vi "Grips Slave UDP (PXI).vi"() -> ()   [LabVIEW 2013]
uses:
  <vilib>/Analysis/Matrix/Datatypes/RealMatrix.ctl
  Telemanipulation/PXI/PXI.lvclass
  Telemanipulation/Grips Robot/Grips Robot.lvclass
  <vilib>/Platform/TimedLoop/XDataNode/timing_clust.ctl
  <vilib>/Platform/TimedLoop/XDataNode/nitl_modes.ctl
  <vilib>/Platform/TimedLoop/XDataNode/wakeup.ctl
  labview_ros/sensor_msgs/JointState.ctl
  labview_ros/std_msgs/Header.ctl
  Telemanipulation/Grips Robot/Grips Robot.lvclass/Grips Robot.ctl
  Telemanipulation/Hardware Interface/Hardware Interface.lvclass/Hardware Interface.ctl
  labview_ros/osrf_msgs/JointCommands.ctl
  Telemanipulation/Hardware Interface/Set HW Interface Analog Outputs.vi
  <userlib>/_matio/level5/Public/Write/Append Data Element.llb/Append Data Element (1D Array of Double).vi
  <userlib>/_matio/level5/Public/Write/Append Data Element.llb/Append Data Element (2D Array of Double).vi
  Telemanipulation/Helpers/Order JointCommands By Name.vi
  <vilib>/addons/control/pid/pid.llb/PID.vi
  <vilib>/addons/control/pid/pid.llb/PID (DBL).vi
  <vilib>/Platform/TimedLoop/XDataNode/XDataNode.xnode
  <vilib>/Platform/TimedLoop/XDataNode/XDNodeRunTimeDep.lvlib
  Telemanipulation/Helpers/Helpers.lvlib
  <userlib>/_matio/level5.lvlib
  <vilib>/Analysis/Matrix/NI_Matrix.lvlib
panel:
  out "end effector transform":T1
  in  "Data Logging":cluster{"Path":path, "Save":bool}={"Path"=path "c:/ni-rt/testing/slave_udp.mat", "Save"=FALSE}
  out "Logging Status":errorcluster
  out "UDP Receiver":cluster{"Rate (Hz)":dbl, "Status":errorcluster}
  out "UDP Sender":cluster{"Rate (Hz)":dbl, "Status":errorcluster}
  out "Joint Names":string[](array[string])=["SA", "SE", "EL", "WP", "WY", "WR"]
  in  "ROS Machine":T2={"IP"="192.168.0.10", "Read Port"=5051, "Write Port"=5052}
  out "WR":dbl(slide)=-0.9473827382931216 scale=-3.14..3.14
  out "WY":dbl(slide)=0.3565705572681916 scale=-1.01..0.67
  out "WP":dbl(slide)=-0.29450757439331093 scale=-1.1..0.58
  out "EL":dbl(slide)=3.229844911017393 scale=0.74..4.2
  out "SE":dbl(slide)=-1.3453457540222367 scale=-1.5..0.5
  out "SA":dbl(slide)=0.31900452488687786 scale=-1.5..1.5
  in  "Hyd ON":bool
  in  "kp_position":dbl[](array[numeric])=[3.0, -1.5, 2.0, 4.0, -2.0, 4.0]
  in  "stop":bool
  out "System Status":errorcluster
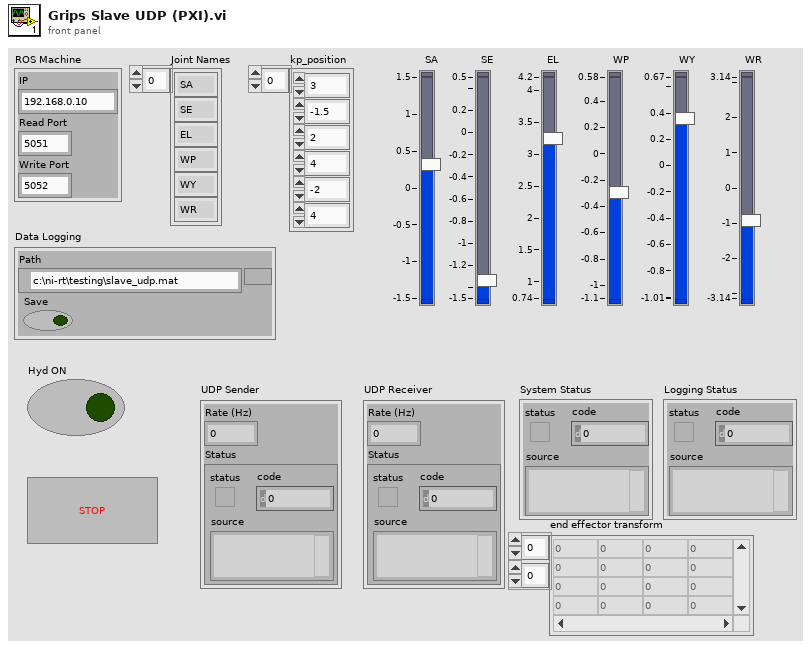
[diagram p1: front panel]
types:
  T1 = typedef "NI_Matrix.lvlib/RealMatrix.ctl" = dbl[][]
  T2 = cluster{"IP":string, "Read Port":u16, "Write Port":u16}
  T3 = typedef "XDNodeRunTimeDep.lvlib/timing_clust.ctl" = cluster{"Expected End [f-1]":u64, "Actual End [f-1]":u64, "Finished Late? [f-1]":bool, "Expected End [i-1]":u64, "Actual End [i-1]":u64, "Finished Late? [i-1]":bool, "Expected Start [i]":u64, "Actual Start [i]":u64, "Expected Start [f]":u64, "Actual Start [f]":u64, "Source Name":string, "Structure Name":string, "Period":i64, "Deadline":i64, "Offset":i64, "Start":i64, "Priority":i32, "Timeout":i32, "Mode":T4, "Wakeup Reason":T5, "Error":errorcluster, "Source Type":string, "Secondary Source Type":string, "Global End Time":u64, "Global Start Time":u64, "Frame Duration":u64, "Iteration Duration":u64, "Assigned CPU":i32, "I/O Scan Engine Mode":u32}
  T4 = typedef "XDNodeRunTimeDep.lvlib/nitl_modes.ctl" = enum32{"No Change", "Process missed periods, maintain original phase", "Discard missed periods, maintain original phase", "Process missed periods, ignore original phase", "Discard missed periods, ignore original phase"}
  T5 = typedef "XDNodeRunTimeDep.lvlib/wakeup.ctl" = enum32{"Normal", "Aborted", "Asynchronous wakeup", "Timing source error", "Timed loop error", "Timeout"}
  T6 = typedef "Grips Robot.lvclass/JointMapping.ctl" = cluster{"name":string[], "position":string[], "velocity":string[], "effort":string[], "command":string[]}
  T7 = cluster{"names":cluster{"AI":string[], "AO":string[], "DI":string[], "DO":string[]}, "interpolation_coeff":sgl[][]}
  T8 = typedef "NI_Robotics_Link.lvclass/Joint Type.ctl" = enum16{"Revolute", "Prismatic"}
  T9 = cluster{"k":sgl[][], "p":sgl[][], "T0":sgl[][], "types":T8[], "joint_limits":cluster{"has_limits":bool[], "min_position":sgl[], "max_position":sgl[]}}
  T10 = enum16{"big-endian, network order", "native, host order", "little-endian"}
  T11 = typedef "JointState.ctl" = cluster{"header":T12, "name":string[], "position":dbl[], "velocity":dbl[], "effort":dbl[]}
  T12 = typedef "Header.ctl" = cluster{"seq":u32, "stamp":cluster{"sec":i32, "nsec":i32}, "frame_id":string}
  T13 = cluster{"seq":u32, "stamp":cluster{"sec":i32, "nsec":i32}, "frame_id":string}
  T14 = cluster{"AI":string[], "AO":string[], "DI":string[], "DO":string[]}
  T15 = typedef "PXI.lvclass/Task Definition.ctl" = cluster{"task_type":T16, "names":string[], "physical channels":tag, "min_value":dbl, "max_value":dbl, "task_number":i32}
  T16 = typedef "PXI.lvclass/Task Types.ctl" = enum16{"Analog Input", "Analog Output", "Digital Input", "Digital Output"}
  T17 = enum16{"open", "replace", "create", "open or create", "replace or create", "replace or create with confirmation"}
  T18 = typedef "Hardware Interface.lvclass/BoolArrayWithName.ctl" = cluster{"name":string[], "value":bool[]}
  T19 = typedef "Hardware Interface.lvclass/DblArrayWithName.ctl" = cluster{"name":string[], "value":dbl[]}
  T20 = typedef "JointCommands.ctl" = cluster{"header":T12, "name":string[], "position":dbl[], "velocity":dbl[], "effort":dbl[], "kp_position":dbl[], "ki_position":dbl[], "kd_position":dbl[], "kp_velocity":dbl[], "i_effort_min":dbl[], "i_effort_max":dbl[]}
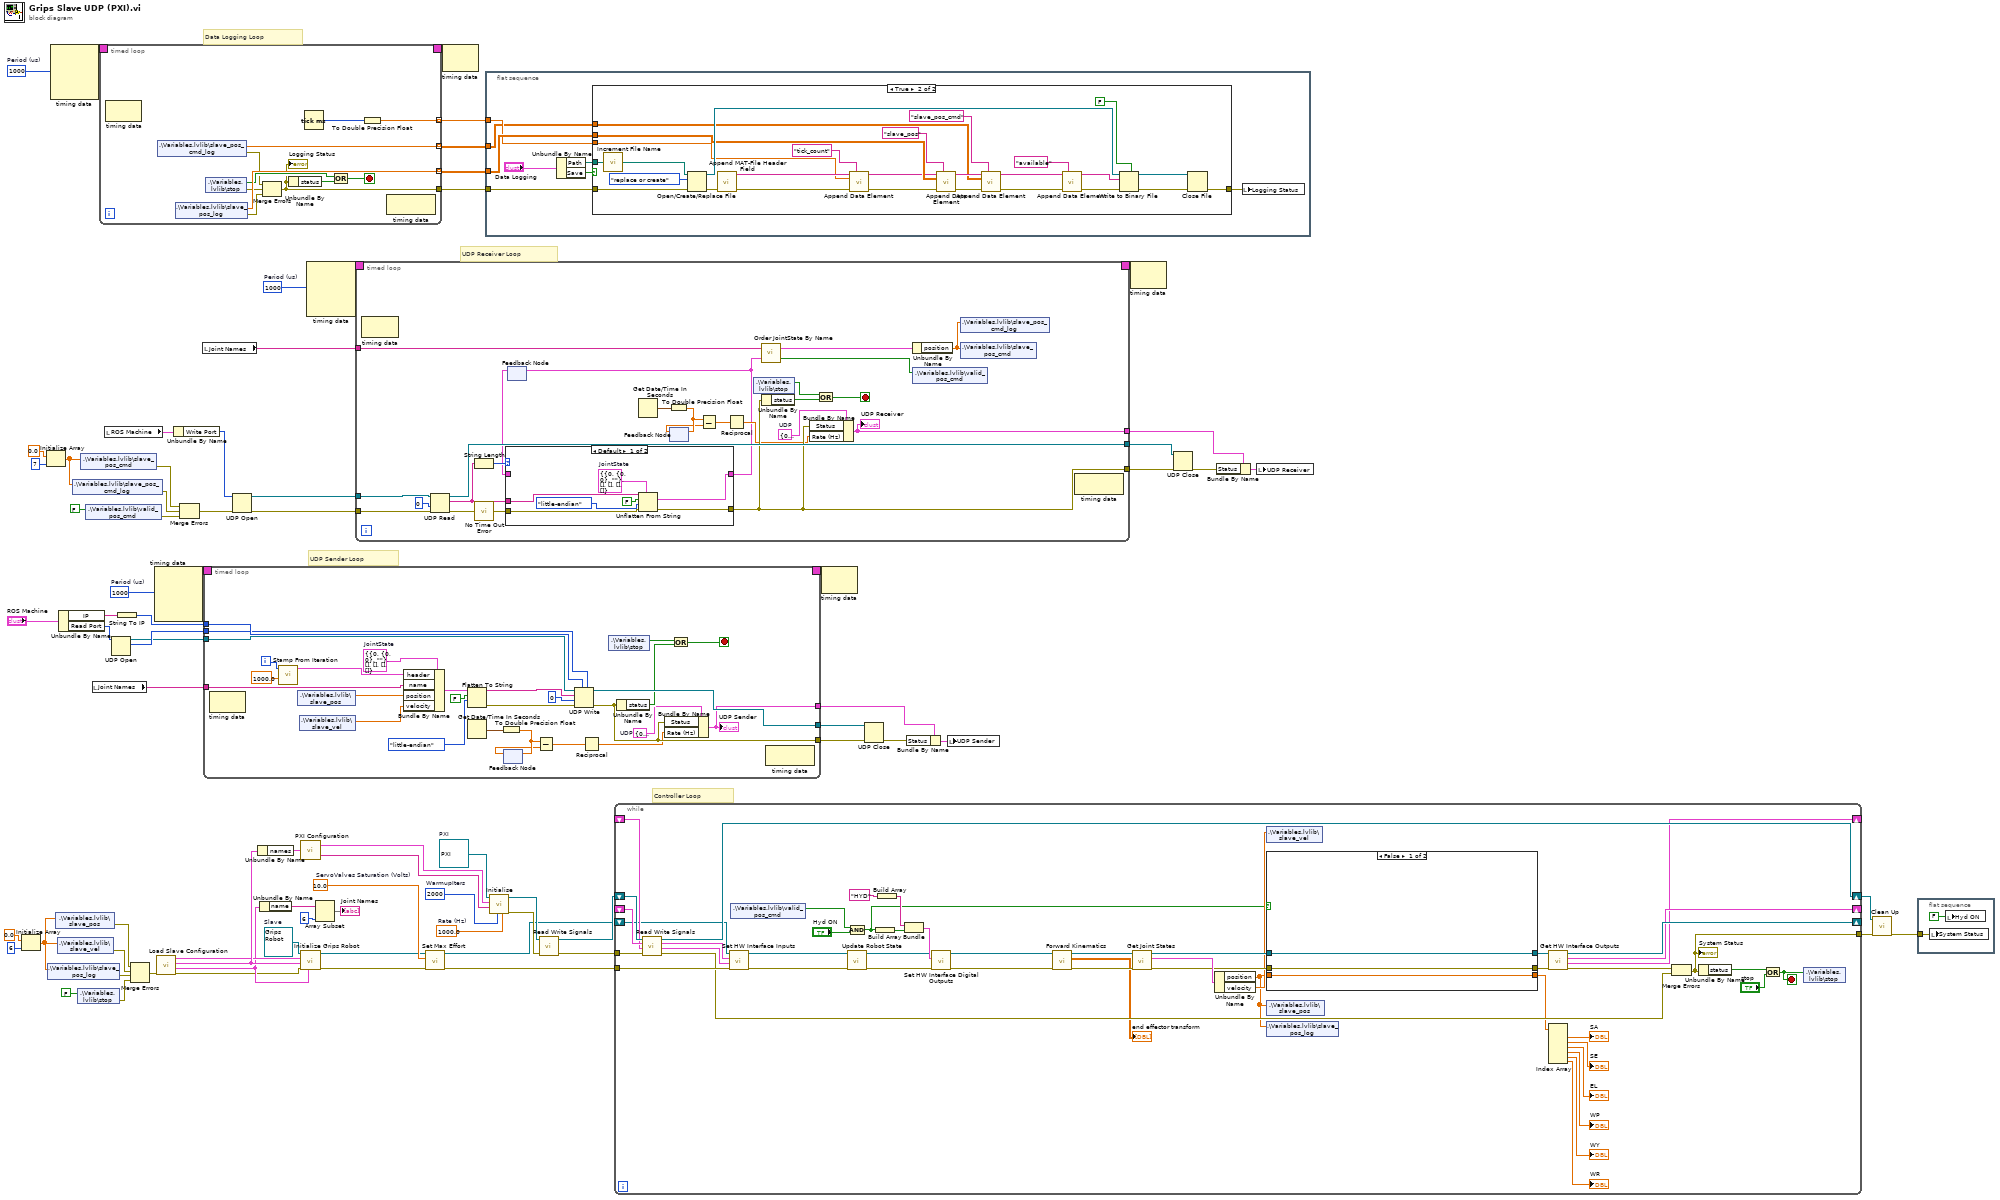
[diagram p0: block diagram]
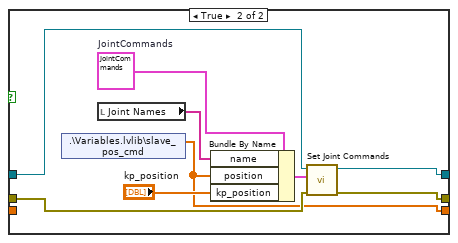
[diagram p4: hidden frame]
diagram:
  w5 = i64 1000  # Period (us)
  w30 = i64 1000  # Period (us)
  w49 = i64 1000  # Period (us)
  w62 = 10.0  # ServoValves Saturation (Volts)
  w65 = refnum<class "Grips Robot.lvclass"> refnum  # Slave
  w76 = 1000.0  # Rate (Hz)
  w77 = u32 2000  # WarmupIters
  w78 = refnum<class "PXI.lvclass"> refnum  # PXI
  # "Data Logging Loop"
  # "Controller Loop"
  # "UDP Receiver Loop"
  # "UDP Sender Loop"
  n1 = Initialize Array(0.0 ("element"), 6 ("dimension size")) -> (w11:dbl[])
  n2 = Initialize Array(0.0 ("element"), 7 ("dimension size")) -> (w2:dbl[])
  n3 = shared-variable ".\\Variables.lvlib\\slave_pos_log"(w11) -> (error out=w10:errorcluster)  [unwired: 1 in]
  n4 = node-c288(w5) -> (w14:T3)  [unwired: 3 in]
  n5 = shared-variable ".\\Variables.lvlib\\slave_pos"(w11) -> (error out=w57:errorcluster)  [unwired: 1 in]
  n6 = shared-variable ".\\Variables.lvlib\\slave_vel"(w11) -> (error out=w56:errorcluster)  [unwired: 1 in]
  n7 = Unbundle By Name("ROS Machine") -> ("IP"=w46:string, "Read Port"=w37:u16)
  n8 = shared-variable ".\\Variables.lvlib\\slave_pos_cmd_log"(w2) -> (error out=w3:errorcluster)  [unwired: 1 in]
  n9 = shared-variable ".\\Variables.lvlib\\stop"(FALSE ("stop")) -> (error out=w9:errorcluster)  [unwired: 1 in]
  n10 = shared-variable ".\\Variables.lvlib\\slave_pos_cmd"(w2) -> (error out=w21:errorcluster)  [unwired: 1 in]
  n11 = shared-variable ".\\Variables.lvlib\\valid_pos_cmd"(FALSE ("valid_pos_cmd")) -> (error out=w4:errorcluster)  [unwired: 1 in]
  n12 = local read "Joint Names"() -> (w38:string[])
  n13 = timed-loop {
    timing: w14 -> [_]
    timing-out: [_] -> w13
    tunnel: [w89] -> w8 mode=indexing
    tunnel: [w87] -> w7 mode=indexing
    tunnel: [w79] -> w6
    tunnel: [w83] -> w1 mode=indexing
    stop <- w84 stop-if-true
    n14 = node-c288() -> ()  [unwired: 1 in, 1 out]
    n15 = shared-variable ".\\Variables.lvlib\\slave_pos_cmd_log"() -> (w83:dbl[], error out=w82:errorcluster)  [unwired: 1 in]
    n16 = shared-variable ".\\Variables.lvlib\\slave_pos_log"() -> (w89:dbl[], error out=w80:errorcluster)  [unwired: 1 in]
    n17 = shared-variable ".\\Variables.lvlib\\stop"() -> (w85:bool, error out=w81:errorcluster)  [unwired: 1 in]
    n18 = Merge Errors(w82, w81, w80) -> (w79:errorcluster)
    "Logging Status" <- w79
    n19 = Unbundle By Name(w79) -> ("status"=w86:bool)
    n20 = Tick Count (ms)() -> (millisecond timer value=w88:u32)
    n21 = Or(x=w85, y=w86) -> (x .or. y?=w84:bool)
    n22 = To Double Precision Float(number=w88) -> (double precision float=w87:dbl)
    n23 = node-c288() -> ()  [unwired: 1 in, 1 out]
  }
  n24 = local read "ROS Machine"() -> (w36:T2)
  n25 = UDP Open(11:w37) -> (port=w43:refnum<k16>, 2:w44:u16)  [unwired: 1 in, 4 out]
  n26 = String To IP(1:w46) -> (0:w45:u32)
  n27 = Merge Errors(w57, w56, w10, w9) -> (w12:errorcluster)
  n28 = node-c288(w49) -> (w51:T3)  [unwired: 3 in]
  n29 = call "Load Slave Configuration.vi"("error in"=w12) -> ("error out"=w33:errorcluster, "JointMapping"=w48:T6, "hw interface"=w64:T7, "kinematic parameters"=w63:T9)  [unwired: 7 in]
  n30 = Unbundle By Name(w36) -> ("Write Port"=w35:u16)
  n31 = Merge Errors(w21, w3, w4) -> (w20:errorcluster)
  n32 = local read "Joint Names"() -> (w22:string[])
  n33 = timed-loop {
    tunnel: [w94] -> w29
    timing: w51 -> [_]
    timing-out: [_] -> w50
    tunnel: w38 -> [w117]
    tunnel: w45 -> [w110]
    tunnel: w44 -> [w109]
    tunnel: w43 -> [w108]
    tunnel: [w106] -> w42
    tunnel: [w92] -> w15
    i -> [w105]
    stop <- w119 stop-if-true
    w95 = cluster{"Rate (Hz)":dbl, "Status":errorcluster} {"Rate (Hz)"=0.0, "Status"={"status"=FALSE, "code"=0, "source"=""}}  # UDP
    w116 = T11 {"header"={"seq"=0, "stamp"={"sec"=0, "nsec"=0}, "frame_id"=""}, "name"=[], "position"=[], "velocity"=[], "effort"=[]}  # JointState
    n34 = node-c288() -> ()  [unwired: 1 in, 1 out]
    n35 = call "Stamp From Iteration.vi"("Rate (Hz)"=1000.0, "Iteration"=w105) -> ("Header"=w103:T13)  [unwired: 9 in]
    n36 = shared-variable ".\\Variables.lvlib\\slave_pos"() -> (w114:dbl[])  [unwired: 1 in, 1 out]
    n37 = shared-variable ".\\Variables.lvlib\\slave_vel"() -> (w115:dbl[])  [unwired: 1 in, 1 out]
    n38 = Bundle By Name(cluster=w116, "header"=w103, "name"=w117, "position"=w114, "velocity"=w115) -> (w118:T11)
    n39 = Flatten To String(anything=w118, prepend array or string size? (T)=FALSE, byte order (0:big-endian, network order)=T10."little-endian") -> (data string=w113:string, error out=w107:errorcluster)  [unwired: 1 in, 1 out]
    n40 = Get Date/Time In Seconds() -> (seconds since 1Jan1904=w100:timestamp)
    n41 = To Double Precision Float(number=w100) -> (double precision float=w101:dbl)
    n42 = feedback #1() -> (w99:dbl)  [unwired: 1 in]
    n43 = feedback-in #1(w101) -> ()
    n44 = Subtract(x=w101, y=w99) -> (x-y=w102:dbl)
    n45 = UDP Write(address=w110, port or service name=w109, connection ID=w108, data in=w113, 8:w107, 9:0 ("timeout ms (25000)")) -> (error out=w94:errorcluster, 3:w106:refnum<k16>)
    n46 = Reciprocal(x=w102) -> (1/x=w93:dbl)
    n47 = shared-variable ".\\Variables.lvlib\\stop"() -> (w96:bool)  [unwired: 1 in, 1 out]
    n48 = Unbundle By Name(w94) -> ("status"=w97:bool)
    n49 = Bundle By Name(cluster=w95, "Status"=w94, "Rate (Hz)"=w93) -> (w92:cluster{"Rate (Hz)":dbl, "Status":errorcluster})
    "UDP Sender" <- w92
    n50 = Or(x=w96, y=w97) -> (x .or. y?=w119:bool)
    n51 = node-c288() -> ()  [unwired: 1 in, 1 out]
  }
  n52 = UDP Open(8:w20, 11:w35) -> (port=w24:refnum<k16>, 0:w23:errorcluster)  [unwired: 4 out]
  n53 = Unbundle By Name(w64) -> ("names"=w66:T14)
  n54 = Unbundle By Name(w48) -> ("name"=w41:string[])
  n55 = call "PXI Configuration.vi"("names"=w66) -> ("Master Clock"=w67:tag, "Tasks Configuration"=w68:T15[])  [unwired: 2 in]
  n56 = call "Initialize Grips Robot.vi"("JointMapping"=w48, "error in (no error)"=w33, "hw interface"=w64, "kinematic_parameters"=w63, "Grips Robot in"=w65) -> ("error out"=w59:errorcluster, "Grips Robot out"=w60:refnum<class "Grips Robot.lvclass">)  [unwired: 5 in]
  n57 = node-c288(w30) -> (w32:T3)  [unwired: 3 in]
  n58 = Array Subset(array=w41, length=6) -> (→"Joint Names":string[])  [unwired: 1 in]
  n59 = timed-loop {
    timing: w32 -> [_]
    timing-out: [_] -> w31
    tunnel: [w131] -> w26
    tunnel: [w140] -> w25
    tunnel: w24 -> [w138]
    tunnel: w23 -> [w137]
    tunnel: w22 -> [w135]
    tunnel: [w125] -> w16
    stop <- w141 stop-if-true
    w132 = cluster{"Rate (Hz)":dbl, "Status":errorcluster} {"Rate (Hz)"=0.0, "Status"={"status"=FALSE, "code"=0, "source"=""}}  # UDP
    n60 = node-c288() -> ()  [unwired: 1 in, 1 out]
    n61 = UDP Read(connection ID=w138, timeout ms (25000)=0 ("timeout (ms)"), 8:w137) -> (data out=w139:string, error out=w144:errorcluster, 3:w140:refnum<k16>)  [unwired: 1 in, 2 out]
    n62 = String Length(string=w139) -> (length=w145:i32)
    n63 = call <vilib>:"No Time Out Error.vi"("error in (no error)"=w144) -> ("error out"=w146:errorcluster)  [unwired: 14 out]
    n64 = feedback #2() -> (w124:T11)  [unwired: 1 in]
    n65 = case shown="Default" w145 {
      tunnel: w139 -> [w152 _]
      tunnel: w146 -> [w151 w155]
      tunnel: [w150 w155] -> w131
      tunnel: [w148 w154] -> w123
      tunnel: w124 -> [_ w154]
      frame Default {
        w147 = T11 {"header"={"seq"=0, "stamp"={"sec"=0, "nsec"=0}, "frame_id"=""}, "name"=[], "position"=[], "velocity"=[], "effort"=[]}  # JointState
        n66 = Unflatten From String(type=w147, binary string=w152, data includes array or string size? (T)=FALSE, byte order (0:big-endian, network order)=T10."little-endian", error in (no error)=w151) -> (value=w148:T11, error out=w150:errorcluster)  [unwired: 1 out]
      }
      frame 0 {
      }
    }
    n67 = feedback-in #2(w123) -> ()
    n68 = Get Date/Time In Seconds() -> (seconds since 1Jan1904=w128:timestamp)
    n69 = To Double Precision Float(number=w128) -> (double precision float=w129:dbl)
    n70 = feedback #3() -> (w127:dbl)  [unwired: 1 in]
    n71 = feedback-in #3(w129) -> ()
    n72 = Subtract(x=w129, y=w127) -> (x-y=w130:dbl)
    n73 = Reciprocal(x=w130) -> (1/x=w126:dbl)
    n74 = shared-variable ".\\Variables.lvlib\\stop"() -> (w143:bool)  [unwired: 1 in, 1 out]
    n75 = call "Order JointState By Name.vi"("JointState In"=w123, "Ordered Joint Names"=w135) -> ("all found?"=w133:bool, "JointState Out"=w134:T11)
    n76 = Unbundle By Name(w131) -> ("status"=w142:bool)
    n77 = Bundle By Name(cluster=w132, "Status"=w131, "Rate (Hz)"=w126) -> (w125:cluster{"Rate (Hz)":dbl, "Status":errorcluster})
    "UDP Receiver" <- w125
    n78 = Or(x=w143, y=w142) -> (x .or. y?=w141:bool)
    n79 = Unbundle By Name(w134) -> ("position"=w122:dbl[])
    n80 = shared-variable ".\\Variables.lvlib\\valid_pos_cmd"(w133) -> ()  [unwired: 1 in, 1 out]
    n81 = shared-variable ".\\Variables.lvlib\\slave_pos_cmd_log"(w122) -> ()  [unwired: 1 in, 1 out]
    n82 = shared-variable ".\\Variables.lvlib\\slave_pos_cmd"(w122) -> ()  [unwired: 1 in, 1 out]
    n83 = node-c288() -> ()  [unwired: 1 in, 1 out]
  }
  n84 = call "Set Max Effort.vi"("error in (no error)"=w59, "max effort"=w62, "Grips Robot in"=w60) -> ("error out"=w61:errorcluster, "Grips Robot out"=w58:refnum<class "Grips Robot.lvclass">)  [unwired: 7 in]
  n85 = node-c288(w13) -> ()  [unwired: 1 out]
  n86 = flat-sequence {
    tunnel: w8 -> [w164]
    tunnel: w7 -> [w163]
    tunnel: w6 -> [w159]
    tunnel: w1 -> [w158]
    frame #0 {
      n87 = Unbundle By Name("Data Logging") -> ("Path"=w161:path, "Save"=w160:bool)
      n88 = case shown="True" w160 {
        tunnel: [w166 w184] -> w165
        tunnel: w164 -> [_ w183]
        tunnel: w163 -> [_ w182]
        tunnel: w161 -> [_ w176]
        tunnel: w159 -> [w166 w178]
        tunnel: w158 -> [_ w173]
        frame False {
        }
        frame True {
          n89 = call "Increment File Name.vi"("Full Path"=w176) -> ("New Path"=w177:path)
          n90 = Open/Create/Replace File(file path (use dialog)=w177, error in=w178, operation (0:open)=T17."replace or create") -> (refnum out=w185:refnum<file>, error out=w181:errorcluster)  [unwired: 3 in, 1 out]
          n91 = call <userlib>:"Append MAT-File Header Field.vi"("error"=w181) -> ("result string"=w189:string, "error out"=w188:errorcluster)  [unwired: 13 in]
          n92 = call-poly <userlib>:"Append Data Element.vi"("initial string"=w189, "Data Name"="tick_count", "data"=w182, "error in"=w188) -> ("result string"=w180:string, "error out"=w179:errorcluster)  [unwired: 10 in]
          n93 = call-poly <userlib>:"Append Data Element.vi"("initial string"=w180, "Data Name"="slave_pos" ("array name"), "data"=w183, "error in"=w179) -> ("result string"=w175:string, "error out"=w174:errorcluster)  [unwired: 10 in]
          n94 = call-poly <userlib>:"Append Data Element.vi"("initial string"=w175, "Data Name"="slave_pos_cmd" ("array name"), "data"=w173, "error in"=w174) -> ("result string"=w168:string, "error out"=w167:errorcluster)  [unwired: 10 in]
          n95 = call-poly <userlib>:"Append Data Element.vi"("initial string"=w168, "Data Name"="available", "error in"=w167) -> ("result string"=w170:string, "error out"=w171:errorcluster)  [unwired: 11 in]
          n96 = Write to Binary File(file (use dialog)=w185, data=w170, error in=w171, 5:FALSE ("prepend array or string size? (T)")) -> (refnum out=w191:refnum<file>, error out=w190:errorcluster)  [unwired: 2 in, 1 out]
          n97 = Close File(refnum=w191, error in=w190) -> (error out=w184:errorcluster)  [unwired: 1 out]
        }
      }
      n98 = local write "Logging Status"(w165) -> ()
    }
  }
  n99 = call "Initialise.vi"("Rate (Hz)"=w76, "WarmupIters"=w77, "Master Clock"=w67, "Tasks Config"=w68, "PXI in"=w78) -> ("error out"=w74:errorcluster, "PXI out"=w75:refnum<class "PXI.lvclass">)  [unwired: 5 in]
  n100 = call "Read Write Signals.vi"("error in (no error)"=w74, "PXI in"=w75) -> ("error out"=w72:errorcluster, "PXI out"=w73:refnum<class "PXI.lvclass">)  [unwired: 6 in, 2 out]
  n101 = while {
    shift-right: [w239] -> w71
    shift-left: w73 -> [w240]
    tunnel: w72 -> [w241]
    tunnel: [w232] -> w70
    tunnel: w61 -> [w236]
    shift-right: [w228] -> _
    shift-left: _ -> [w229]
    shift-right: [w226] -> _
    shift-left: _ -> [w227]
    shift-right: [w235] -> _
    shift-left: w58 -> [w212]
    stop <- w211 stop-if-true
    n102 = call "Read Write Signals.vi"("error in (no error)"=w241, "Digital Outputs"=w227, "Analog Outputs"=w229, "PXI in"=w240) -> ("error out"=w233:errorcluster, "Digital Inputs"=w230:T18, "Analog Inputs"=w231:T19, "PXI out"=w239:refnum<class "PXI.lvclass">)  [unwired: 4 in]
    n103 = call "Set HW Interface Inputs.vi"("error in (no error)"=w236, "Digital Inputs"=w230, "Analog Inputs"=w231, "Grips Robot in"=w212) -> ("error out"=w224:errorcluster, "Grips Robot out"=w225:refnum<class "Grips Robot.lvclass">)  [unwired: 6 in]
    n104 = shared-variable ".\\Variables.lvlib\\valid_pos_cmd"() -> (w200:bool)  [unwired: 1 in, 1 out]
    n105 = And(x=w200, y="Hyd ON") -> (x .and. y?=w199:bool)
    n106 = call "Update Robot State.vi"("error in (no error)"=w224, "Grips Robot in"=w225) -> ("error out"=w213:errorcluster, "Grips Robot out"=w214:refnum<class "Grips Robot.lvclass">)  [unwired: 8 in]
    n107 = Build Array(w199) -> (w217:bool[])
    n108 = Build Array("HYD") -> (w216:string[])
    n109 = Bundle(w216, w217) -> (w218:cluster{string[], bool[]})  [unwired: 1 in]
    n110 = call "Set HW Interface Digital Outputs.vi"("error in (no error)"=w213, "Digital Outputs"=w218, "Grips Robot in"=w214) -> ("error out"=w195:errorcluster, "Grips Robot out"=w196:refnum<class "Grips Robot.lvclass">)  [unwired: 7 in]
    n111 = call "Forward Kinematics.vi"("error in (no error)"=w195, "Grips Robot in"=w196) -> ("error out"=w198:errorcluster, "end effector transform"=→"end effector transform":T1, "Grips Robot out"=w197:refnum<class "Grips Robot.lvclass">)  [unwired: 7 in]
    n112 = call "Get Joint States.vi"("error in (no error)"=w198, "Grips Robot in"=w197) -> ("error out"=w220:errorcluster, "JointState"=w223:T11, "Grips Robot out"=w222:refnum<class "Grips Robot.lvclass">)  [unwired: 7 in]
    n113 = Unbundle By Name(w223) -> ("position"=w209:dbl[], "velocity"=w210:dbl[])
    n114 = shared-variable ".\\Variables.lvlib\\slave_vel"(w210) -> ()  [unwired: 1 in, 1 out]
    n115 = case shown="False" w199 {
      tunnel: w209 -> [w242 _]
      tunnel: w222 -> [w244 w248]
      tunnel: [w244 w252] -> w221
      tunnel: w220 -> [w243 w251]
      tunnel: [w243 w250] -> w219
      tunnel: [w242 w246] -> w202
      frame False {
      }
      frame True {
        w245 = T20 {"header"={"seq"=0, "stamp"={"sec"=0, "nsec"=0}, "frame_id"=""}, "name"=[], "position"=[], "velocity"=[], "effort"=[], "kp_position"=[], "ki_position"=[], "kd_position"=[], "kp_velocity"=[], "i_effort_min"=[], "i_effort_max"=[]}  # JointCommands
        n116 = shared-variable ".\\Variables.lvlib\\slave_pos_cmd"() -> (w246:dbl[])  [unwired: 1 in, 1 out]
        n117 = local read "Joint Names"() -> (w247:string[])
        n118 = Bundle By Name(cluster=w245, "name"=w247, "position"=w246, "kp_position"="kp_position") -> (w253:T20)
        n119 = call "Set Joint Commands.vi"("error in (no error)"=w251, "JointCommands"=w253, "Grips Robot in"=w248) -> ("error out"=w250:errorcluster, "Grips Robot out"=w252:refnum<class "Grips Robot.lvclass">)  [unwired: 7 in]
      }
    }
    n120 = shared-variable ".\\Variables.lvlib\\slave_pos"(w209) -> ()  [unwired: 1 in, 1 out]
    n121 = shared-variable ".\\Variables.lvlib\\slave_pos_log"(w209) -> ()  [unwired: 1 in, 1 out]
    n122 = call "Get HW Interface Outputs.vi"("error in (no error)"=w219, "Grips Robot in"=w221) -> ("error out"=w234:errorcluster, "Digital Outputs"=w226:T18, "Analog Outputs"=w228:T19, "Grips Robot out"=w235:refnum<class "Grips Robot.lvclass">)  [unwired: 6 in]
    n123 = Index Array(array=w202) -> (element #1=→"SA":dbl, element #2=→"SE":dbl, element #3=→"EL":dbl, element #4=→"WP":dbl, element #5=→"WY":dbl, element #6=→"WR":dbl)  [unwired: 6 in]
    n124 = Merge Errors(w234, w233) -> (w232:errorcluster)
    "System Status" <- w232
    n125 = Unbundle By Name(w232) -> ("status"=w238:bool)
    n126 = Or(x=w238, y="stop") -> (x .or. y?=w211:bool)
    n127 = shared-variable ".\\Variables.lvlib\\stop"(w211) -> ()  [unwired: 1 in, 1 out]
  }
  n128 = node-c288(w50) -> ()  [unwired: 1 out]
  n129 = UDP Close(connection ID=w42, 8:w29) -> (error out=w28:errorcluster)  [unwired: 1 out]
  n130 = Bundle By Name(cluster=w15, "Status"=w28) -> (w27:cluster{"Rate (Hz)":dbl, "Status":errorcluster})
  n131 = local write "UDP Sender"(w27) -> ()
  n132 = node-c288(w31) -> ()  [unwired: 1 out]
  n133 = UDP Close(connection ID=w25, 8:w26) -> (error out=w17:errorcluster)  [unwired: 1 out]
  n134 = Bundle By Name(cluster=w16, "Status"=w17) -> (w18:cluster{"Rate (Hz)":dbl, "Status":errorcluster})
  n135 = local write "UDP Receiver"(w18) -> ()
  n136 = call "Clean Up.vi"("error in (no error)"=w70, "PXI in"=w71) -> ("error out"=w69:errorcluster)  [unwired: 8 in, 1 out]
  n137 = flat-sequence {
    tunnel: w69 -> [w255]
    frame #0 {
      n138 = local write "System Status"(w255) -> ()
      n139 = local write "Hyd ON"(FALSE ("Hyd ON")) -> ()
    }
  }
